vi "Dashboard custom_bartender&global&gripper.vi"() -> ()   [LabVIEW 2017]
uses:
  C:/Users/IMR Lab/Documents/LabVIEW Data/UniversalRobotsSDK_LABView/LabVIEW/Examples/LabVIEW10/UnderAutomation.UniversalRobots.dll
  UnderAutomation.UniversalRobots.dll
  Global 1.vi
panel:
  out "3rd Order":bool
  out "2nd Order":bool
  out "1st Order":bool
  in  "stop":bool
  in  "TCP switch (server)":bool
  out "Rx":dbl
  out "Rz":dbl
  out "Ry":dbl
  out "Enabled":bool
  out "Port":i32
  in  "Move to particular posture":bool
  in  "Move to Zero position":bool
  out "Connected":bool
  in  "Robot IP(192.168.112.182)":string
  out "Connect error":errorcluster
  in  "Power on\nRelease brake":bool
  in  "Power off":bool
  in  "Connect":bool
  in  "Send script":bool
  in  "Script to execute":string
  out "Powered on":bool
  out "X":dbl
  out "Y":dbl
  out "Z":dbl
  out "License state":string
  # "movel(p[-0.0753945, -0.304532, 0.314608, -0.194623, 2.71667, -1.00228], a= 0.5, v=0.25)"
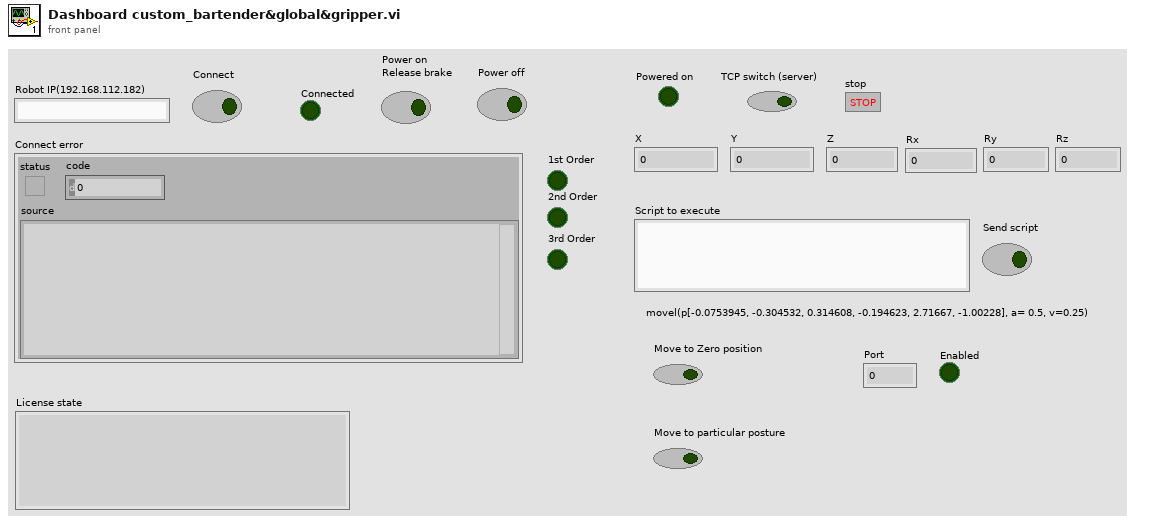
[diagram p1: front panel]
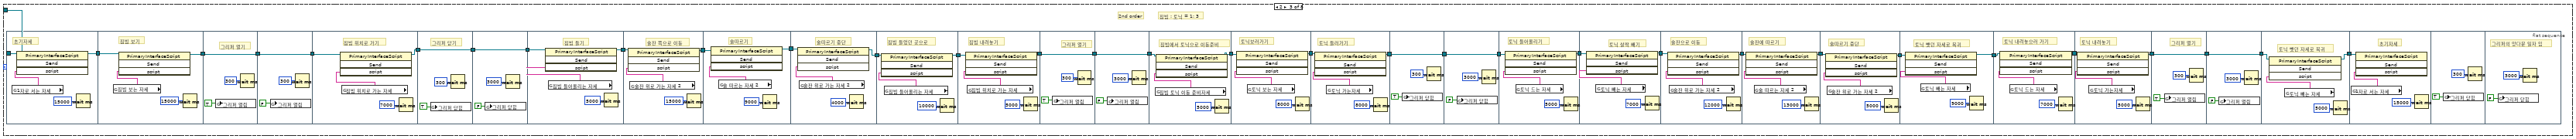
[diagram p5: hidden frame]
diagram:
  # "미니콜라 따르는 자세"
  # "술잔 중간지점 가는 자세"
  # "짐빔에서 토닉이동 준비 자세"
  # "술잔 따르는 자세2"
  # "술잔 위로 가는 자세2"
  # "토닉워터 뺴는 자세"
  # "토닉워 들어올리는 자세"
  # "토닉워터 가는 자세"
  # "토닉워터 보는 자세"
  # "짐빔 들어올리는 자세"
  # "짐빔로 가는 자세"
  # "짐빔 보는 자세"
  # "콜라 뺴는 자세"
  # "콜라 들어올리는 자세"
  # "콜라로 가는 자세"
  # "콜라 보는 자세"
  # "술잔 따르는 자세"
  # "술잔 위로 가는 자세"
  # "잭다니엘 들어올리는 자세"
  # "잭다니엘 위치로 가는 자세"
  # "잭다니엘 보는 자세"
  # "1자로 서는 자세"
  # "Example : Display power on status"
  # "Create a UR\ncobot instance"
  # "Show license state"
  # "Register your confidential license key to exit\ntrial period and use this library forever"
  # "Power off when button is clicked"
  # "Power on and release brake when button is clicked"
  # "Get your UR Dashboard interface"
  n1 = global write "Global 1.vi" "미니콜라 따르는 자세"("movej([-0.0902,-1.8120,-1.9241,-3.5769,6.2827,8.4658], a=0.5, v=0.25, t=0, r=0)") -> ()
  n2 = global write "Global 1.vi" "술잔 중간지점"("movej([-0.2173,-1.9485,-1.6874,-3.9352,6.2671,7.2276], a=0.5, v=0.25, t=0, r=0)") -> ()
  n3 = global write "Global 1.vi" "짐빔 토닉 이동 준비자세"("movej([-0.5421,-0.8131,0.8439,-0.0538,2.5052,5.9032], a=0.5, v=0.25, t=0, r=0)") -> ()
  n4 = global write "Global 1.vi" "잭다니엘 들어올리는 자세"("movej([0.8116,-2.0223,-1.2828,-3.0107,4.3284,5.9341], a=0.5, v=0.25, t=0, r=0)") -> ()
  n5 = global write "Global 1.vi" "잭다닐 위치로 가는 자세"("movej([0.8116,-2.3119,-1.606,-2.3958,4.3284,5.9341], a=0.5, v=0.25, t=0, r=0)") -> ()
  n6 = global write "Global 1.vi" "짐빔 들어올리는 자세"("movej([-0.5421,-0.8131,0.8439,-0.0538,2.5052,5.9032], a=0.5, v=0.25, t=0, r=0)") -> ()
  n7 = global write "Global 1.vi" "술잔 위로 가는 자세 2"("movej([0.0485,-1.6015,2.5780,-1.0382,-0.0520,5.3649], a=0.5, v=0.25, t=0, r=0)") -> ()
  n8 = global write "Global 1.vi" "1자로 서는 자세"("movej([3.1412,-1.5708,0,-1.5708,3.1412,5.8904], a=0.5, v=0.25, t=0, r=0)") -> ()
  n9 = global write "Global 1.vi" "짐빔 위치로 가는 자세"("movej([-0.5436,-0.4519,0.8428,-0.3534,2.6134,5.9032], a=0.5, v=0.25, t=0, r=0)") -> ()
  n10 = global write "Global 1.vi" "술잔 위로 가는 자세"("movej([-0.0903,-2.0548,-2.0169,-3.3289,6.2826,7.4091], a=0.5, v=0.25, t=0, r=0)") -> ()
  n11 = global write "Global 1.vi" "잭다니엘 보는 자세"("movej([0,-2.2170,-1.4226,-2.2842,3.1412,6.2832], a=0.5, v=0.25, t=0, r=0)") -> ()
  n12 = global write "Global 1.vi" "콜라 빼는 자세"("movej([0.8789,-1.5237,-2.1070,-2.6679, 3.9917,5.9085], a=0.5, v=0.25, t=0, r=0)") -> ()
  n13 = global write "Global 1.vi" "콜라 드는 자세"("movej([1.2020,-1.8452,-1.7403,-2.7082,4.3162,5.9158], a=0.5, v=0.25, t=0, r=0)") -> ()
  n14 = global write "Global 1.vi" "콜라 보는 자세"("movej([0,-1.8110,-2.1684,-2.3033,3.1543,5.9213], a=0.5, v=0.25, t=0, r=0)") -> ()
  n15 = global write "Global 1.vi" "콜라로 가는자세"("movej([1.2020,-2.166,-1.9385,-2.1863,4.3172,5.9210], a=0.5, v=0.25, t=0, r=0)") -> ()
  n16 = global write "Global 1.vi" "토닉 빼는 자세"("movej([-0.5277,-1.5104,1.5889,-0.0548,2.5728,5.9025], a=0.5, v=0.25, t=0, r=0)") -> ()
  n17 = global write "Global 1.vi" "술 따르는 자세 2"("movej([0.0412,-1.9708,2.4700,-1.0157,-0.0618,4.8998], a=0.5, v=0.25, t=0, r=0)") -> ()
  n18 = global write "Global 1.vi" "짐빔 보는 자세"("movej([-0.0364,-0.6154,0.9421,-0.3291,3.1047,5.9020], a=0.5, v=0.25, t=0, r=0)") -> ()
  n19 = global write "Global 1.vi" "토닉 드는 자세"("movej([-1.0311,-1.1460,1.5830,-0.4348,2.0708,5.9048], a=0.5, v=0.25, t=0, r=0)") -> ()
  n20 = global write "Global 1.vi" "토닉 보는 자세"("movej([-0.4690,-1.1292,2.1508,-1.0119,2.6124,5.9032], a=0.5, v=0.25, t=0, r=0)") -> ()
  n21 = global write "Global 1.vi" "술 따르는 자세"("movej([-0.0902,-1.9024,-1.9241,-3.5769,6.2827,8.4692], a=0.5, v=0.25, t=0, r=0)") -> ()
  n22 = global write "Global 1.vi" "토닉 가는자세"("movej([-0.9924,-0.8742,1.7459,-0.8837,2.0958,5.9048], a=0.5, v=0.25, t=0, r=0)") -> ()
  n23 = constructor class="UR"() -> (reference out=w25:refnum<k24>)  [unwired: 3 in, 2 out]
  n24 = while {
    tunnel: w25 -> [w31]
    stop <- FALSE stop-if-true
    # "Connect to the robot when button is pressed"
    # "Show if primary interface is connected"
    # "Get your UR primary interface"
    n25 = property class="UR"(reference=w31) -> ("PrimaryInterface"=w34:refnum<k24>)  [unwired: 1 in, 2 out]
    n26 = Wait (ms)(milliseconds to wait=u32 50) -> ()  [unwired: 1 out]
    n27 = property class="PrimaryInterfaceClientInternal"(reference=w34) -> ("Connected"=w33:bool)  [unwired: 1 in, 2 out]
    "Connected" <- w33
    n28 = case shown="True" "Connect" {
      tunnel: w31 -> [_ w397]
      frame False {
      }
      frame True {
        n29 = flat-sequence {
          tunnel: w397 -> [w399]
          frame #0 {
            n30 = invoke class="UR" method="Connect"(reference=w399, "ip"="Robot IP(192.168.112.182)") -> (error out=→"Connect error":errorcluster)  [unwired: 2 in, 3 out]
          }
        }
      }
    }
    n31 = case shown="True" w33 {
      tunnel: w34 -> [_ w55]
      frame False {
      }
      frame True {
        # "Send URScript when button pressed"
        # "Example : Display current cartesian pose"
        n32 = property class="PrimaryInterfaceClientInternal"(reference=w55) -> ("Script"=w40:refnum<k24>)  [unwired: 1 in, 2 out]
        n33 = global read "Global 1.vi" "2nd Order"() -> (w43:bool)
        "2nd Order" <- w43
        n34 = global read "Global 1.vi" "3rd Order"() -> (w42:bool)
        "3rd Order" <- w42
        n35 = global read "Global 1.vi" "1st Order"() -> (w44:bool)
        "1st Order" <- w44
        n36 = Build Array(w44, w43, w42) -> (w45:bool[])
        n37 = Boolean Array To Number(Boolean array=w45) -> (number=w41:u32)
        n38 = case shown="1" w41 {
          tunnel: w40 -> [_ w96 w232 _ _ _ _ _]
          frame 0, Default {
          }
          frame 1 {
            # "잭다 : 콜라 = 1 : 3"
            # "1st order"
            n39 = flat-sequence {
              tunnel: w96 -> [w100]
              tunnel: [w99] -> w95
              tunnel: w95 -> [w104]
              tunnel: [w102] -> w87
              tunnel: w87 -> [w107]
              tunnel: [w107] -> w85
              tunnel: w85 -> [w110]
              tunnel: [w110] -> w84
              tunnel: w84 -> [w114]
              tunnel: [w111] -> w86
              tunnel: w86 -> [w117]
              tunnel: [w117] -> w83
              tunnel: w83 -> [w120]
              tunnel: [w120] -> w82
              tunnel: w82 -> [w122]
              tunnel: [w121] -> w69
              tunnel: w69 -> [w126]
              tunnel: [w125] -> w68
              tunnel: w68 -> [w130]
              tunnel: [w129] -> w94
              tunnel: w94 -> [w135]
              tunnel: [w133] -> w93
              tunnel: w93 -> [w138]
              tunnel: [w137] -> w67
              tunnel: w67 -> [w142]
              tunnel: [w141] -> w66
              tunnel: [w145] -> w92
              tunnel: w66 -> [w147]
              tunnel: w92 -> [w150]
              tunnel: [w149] -> w81
              tunnel: w81 -> [w155]
              tunnel: [w155] -> w80
              tunnel: w80 -> [w158]
              tunnel: [w158] -> w79
              tunnel: w79 -> [w160]
              tunnel: [w159] -> w91
              tunnel: w91 -> [w164]
              tunnel: [w163] -> w78
              tunnel: w78 -> [w169]
              tunnel: [w169] -> w77
              tunnel: w77 -> [w172]
              tunnel: [w172] -> w76
              tunnel: w76 -> [w174]
              tunnel: [w173] -> w75
              tunnel: w75 -> [w178]
              tunnel: [w177] -> w65
              tunnel: w65 -> [w182]
              tunnel: [w181] -> w64
              tunnel: w64 -> [w186]
              tunnel: [w185] -> w90
              tunnel: w90 -> [w190]
              tunnel: [w189] -> w89
              tunnel: w89 -> [w194]
              tunnel: [w193] -> w63
              tunnel: w63 -> [w198]
              tunnel: [w197] -> w62
              tunnel: w62 -> [w202]
              tunnel: [w201] -> w74
              tunnel: w74 -> [w206]
              tunnel: [w205] -> w88
              tunnel: w88 -> [w210]
              tunnel: [w209] -> w72
              tunnel: [w213] -> w73
              tunnel: w72 -> [w213]
              tunnel: [w216] -> w71
              tunnel: w73 -> [w216]
              tunnel: w71 -> [w220]
              tunnel: [w219] -> w70
              tunnel: w70 -> [w223]
              frame #0 {
                # "초기자세"
                n40 = global read "Global 1.vi" "1자로 서는 자세"() -> (w98:string)
                n41 = invoke class="PrimaryInterfaceScript" method="Send"(reference=w100, "script"=w98) -> (reference out=w99:refnum<k24>)  [unwired: 2 in, 3 out]
                n42 = Wait (ms)(milliseconds to wait=u32 15000) -> ()  [unwired: 1 out]
              }
              frame #1 {
                # "잭다니엘 보기"
                n43 = global read "Global 1.vi" "잭다니엘 보는 자세"() -> (w103:string)
                n44 = invoke class="PrimaryInterfaceScript" method="Send"(reference=w104, "script"=w103) -> (reference out=w102:refnum<k24>)  [unwired: 2 in, 3 out]
                n45 = Wait (ms)(milliseconds to wait=u32 15000) -> ()  [unwired: 1 out]
              }
              frame #2 {
                # "그리퍼 열기"
                n46 = global write "Global 1.vi" "그리퍼 열림"(TRUE ("그리퍼 열림")) -> ()
                n47 = Wait (ms)(milliseconds to wait=u32 300) -> ()  [unwired: 1 out]
              }
              frame #3 {
                n48 = global write "Global 1.vi" "그리퍼 열림"(FALSE ("그리퍼 열림")) -> ()
                n49 = Wait (ms)(milliseconds to wait=u32 300) -> ()  [unwired: 1 out]
              }
              frame #4 {
                # "잭다니엘 위치로 가기"
                n50 = global read "Global 1.vi" "잭다닐 위치로 가는 자세"() -> (w113:string)
                n51 = invoke class="PrimaryInterfaceScript" method="Send"(reference=w114, "script"=w113) -> (reference out=w111:refnum<k24>)  [unwired: 2 in, 3 out]
                n52 = Wait (ms)(milliseconds to wait=u32 7000) -> ()  [unwired: 1 out]
              }
              frame #5 {
                # "그리퍼 닫기"
                n53 = global write "Global 1.vi" "그리퍼 닫힘"(TRUE ("그리퍼 열림")) -> ()
                n54 = Wait (ms)(milliseconds to wait=u32 300) -> ()  [unwired: 1 out]
              }
              frame #6 {
                n55 = global write "Global 1.vi" "그리퍼 닫힘"(FALSE ("그리퍼 열림")) -> ()
                n56 = Wait (ms)(milliseconds to wait=u32 3000) -> ()  [unwired: 1 out]
              }
              frame #7 {
                # "잭다니엘 들기"
                n57 = global read "Global 1.vi" "잭다니엘 들어올리는 자세"() -> (w124:string)
                n58 = invoke class="PrimaryInterfaceScript" method="Send"(reference=w122, "script"=w124) -> (reference out=w121:refnum<k24>)  [unwired: 2 in, 3 out]
                n59 = Wait (ms)(milliseconds to wait=u32 3000) -> ()  [unwired: 1 out]
              }
              frame #8 {
                # "술잔 중간지점으로 이동"
                n60 = global read "Global 1.vi" "술잔 중간지점"() -> (w127:string)
                n61 = invoke class="PrimaryInterfaceScript" method="Send"(reference=w126, "script"=w127) -> (reference out=w125:refnum<k24>)  [unwired: 2 in, 3 out]
                n62 = Wait (ms)(milliseconds to wait=u32 15000) -> ()  [unwired: 1 out]
              }
              frame #9 {
                # "술잔 쪽으로 이동"
                n63 = global read "Global 1.vi" "술잔 위로 가는 자세"() -> (w131:string)
                n64 = invoke class="PrimaryInterfaceScript" method="Send"(reference=w130, "script"=w131) -> (reference out=w129:refnum<k24>)  [unwired: 2 in, 3 out]
                n65 = Wait (ms)(milliseconds to wait=u32 5000) -> ()  [unwired: 1 out]
              }
              frame #10 {
                # "술따르기"
                n66 = global read "Global 1.vi" "술 따르는 자세"() -> (w134:string)
                n67 = invoke class="PrimaryInterfaceScript" method="Send"(reference=w135, "script"=w134) -> (reference out=w133:refnum<k24>)  [unwired: 2 in, 3 out]
                n68 = Wait (ms)(milliseconds to wait=u32 9000) -> ()  [unwired: 1 out]
              }
              frame #11 {
                # "술따르기 중단"
                n69 = global read "Global 1.vi" "술잔 위로 가는 자세"() -> (w139:string)
                n70 = invoke class="PrimaryInterfaceScript" method="Send"(reference=w138, "script"=w139) -> (reference out=w137:refnum<k24>)  [unwired: 2 in, 3 out]
                n71 = Wait (ms)(milliseconds to wait=u32 4000) -> ()  [unwired: 1 out]
              }
              frame #12 {
                # "술잔 중간지점으로 이동"
                n72 = global read "Global 1.vi" "술잔 중간지점"() -> (w143:string)
                n73 = invoke class="PrimaryInterfaceScript" method="Send"(reference=w142, "script"=w143) -> (reference out=w141:refnum<k24>)  [unwired: 2 in, 3 out]
                n74 = Wait (ms)(milliseconds to wait=u32 7000) -> ()  [unwired: 1 out]
              }
              frame #13 {
                # "잭다니엘 들었던 곳으로"
                n75 = global read "Global 1.vi" "잭다니엘 들어올리는 자세"() -> (w146:string)
                n76 = invoke class="PrimaryInterfaceScript" method="Send"(reference=w147, "script"=w146) -> (reference out=w145:refnum<k24>)  [unwired: 2 in, 3 out]
                n77 = Wait (ms)(milliseconds to wait=u32 10000) -> ()  [unwired: 1 out]
              }
              frame #14 {
                # "잭다니엘 내려놓기"
                n78 = global read "Global 1.vi" "잭다닐 위치로 가는 자세"() -> (w152:string)
                n79 = invoke class="PrimaryInterfaceScript" method="Send"(reference=w150, "script"=w152) -> (reference out=w149:refnum<k24>)  [unwired: 2 in, 3 out]
                n80 = Wait (ms)(milliseconds to wait=u32 5000) -> ()  [unwired: 1 out]
              }
              frame #15 {
                # "그리퍼 열기"
                n81 = global write "Global 1.vi" "그리퍼 열림"(TRUE ("그리퍼 열림")) -> ()
                n82 = Wait (ms)(milliseconds to wait=u32 300) -> ()  [unwired: 1 out]
              }
              frame #16 {
                n83 = global write "Global 1.vi" "그리퍼 열림"(FALSE ("그리퍼 열림")) -> ()
                n84 = Wait (ms)(milliseconds to wait=u32 3000) -> ()  [unwired: 1 out]
              }
              frame #17 {
                # "콜라보러가기"
                n85 = global read "Global 1.vi" "콜라 보는 자세"() -> (w162:string)
                n86 = invoke class="PrimaryInterfaceScript" method="Send"(reference=w160, "script"=w162) -> (reference out=w159:refnum<k24>)  [unwired: 2 in, 3 out]
                n87 = Wait (ms)(milliseconds to wait=u32 8000) -> ()  [unwired: 1 out]
              }
              frame #18 {
                # "콜라 들러가기"
                n88 = global read "Global 1.vi" "콜라로 가는자세"() -> (w166:string)
                n89 = invoke class="PrimaryInterfaceScript" method="Send"(reference=w164, "script"=w166) -> (reference out=w163:refnum<k24>)  [unwired: 2 in, 3 out]
                n90 = Wait (ms)(milliseconds to wait=u32 8000) -> ()  [unwired: 1 out]
              }
              frame #19 {
                n91 = global write "Global 1.vi" "그리퍼 닫힘"(TRUE ("그리퍼 열림")) -> ()
                n92 = Wait (ms)(milliseconds to wait=u32 300) -> ()  [unwired: 1 out]
              }
              frame #20 {
                n93 = global write "Global 1.vi" "그리퍼 닫힘"(FALSE ("그리퍼 열림")) -> ()
                n94 = Wait (ms)(milliseconds to wait=u32 3000) -> ()  [unwired: 1 out]
              }
              frame #21 {
                # "콜라 들어올리기"
                n95 = global read "Global 1.vi" "콜라 드는 자세"() -> (w176:string)
                n96 = invoke class="PrimaryInterfaceScript" method="Send"(reference=w174, "script"=w176) -> (reference out=w173:refnum<k24>)  [unwired: 2 in, 3 out]
                n97 = Wait (ms)(milliseconds to wait=u32 5000) -> ()  [unwired: 1 out]
              }
              frame #22 {
                # "콜라 살짝 빼기"
                n98 = global read "Global 1.vi" "콜라 빼는 자세"() -> (w180:string)
                n99 = invoke class="PrimaryInterfaceScript" method="Send"(reference=w178, "script"=w180) -> (reference out=w177:refnum<k24>)  [unwired: 2 in, 3 out]
                n100 = Wait (ms)(milliseconds to wait=u32 5000) -> ()  [unwired: 1 out]
              }
              frame #23 {
                # "술잔 중간지점으로 이동"
                n101 = global read "Global 1.vi" "술잔 중간지점"() -> (w183:string)
                n102 = invoke class="PrimaryInterfaceScript" method="Send"(reference=w182, "script"=w183) -> (reference out=w181:refnum<k24>)  [unwired: 2 in, 3 out]
                n103 = Wait (ms)(milliseconds to wait=u32 15000) -> ()  [unwired: 1 out]
              }
              frame #24 {
                # "술잔으로 이동"
                n104 = global read "Global 1.vi" "술잔 위로 가는 자세"() -> (w188:string)
                n105 = invoke class="PrimaryInterfaceScript" method="Send"(reference=w186, "script"=w188) -> (reference out=w185:refnum<k24>)  [unwired: 2 in, 3 out]
                n106 = Wait (ms)(milliseconds to wait=u32 5000) -> ()  [unwired: 1 out]
              }
              frame #25 {
                # "미니콜라에 따르기"
                n107 = global read "Global 1.vi" "미니콜라 따르는 자세"() -> (w192:string)
                n108 = invoke class="PrimaryInterfaceScript" method="Send"(reference=w190, "script"=w192) -> (reference out=w189:refnum<k24>)  [unwired: 2 in, 3 out]
                n109 = Wait (ms)(milliseconds to wait=u32 11000) -> ()  [unwired: 1 out]
              }
              frame #26 {
                # "술따르기 중단"
                n110 = global read "Global 1.vi" "술잔 위로 가는 자세"() -> (w196:string)
                n111 = invoke class="PrimaryInterfaceScript" method="Send"(reference=w194, "script"=w196) -> (reference out=w193:refnum<k24>)  [unwired: 2 in, 3 out]
                n112 = Wait (ms)(milliseconds to wait=u32 5000) -> ()  [unwired: 1 out]
              }
              frame #27 {
                # "술잔 중간지점으로 이동"
                n113 = global read "Global 1.vi" "술잔 중간지점"() -> (w199:string)
                n114 = invoke class="PrimaryInterfaceScript" method="Send"(reference=w198, "script"=w199) -> (reference out=w197:refnum<k24>)  [unwired: 2 in, 3 out]
                n115 = Wait (ms)(milliseconds to wait=u32 7000) -> ()  [unwired: 1 out]
              }
              frame #28 {
                # "콜라 뻇던 자세로 복귀"
                n116 = global read "Global 1.vi" "콜라 빼는 자세"() -> (w203:string)
                n117 = invoke class="PrimaryInterfaceScript" method="Send"(reference=w202, "script"=w203) -> (reference out=w201:refnum<k24>)  [unwired: 2 in, 3 out]
                n118 = Wait (ms)(milliseconds to wait=u32 7000) -> ()  [unwired: 1 out]
              }
              frame #29 {
                # "콜라 내려놓으러 가기"
                n119 = global read "Global 1.vi" "콜라 드는 자세"() -> (w208:string)
                n120 = invoke class="PrimaryInterfaceScript" method="Send"(reference=w206, "script"=w208) -> (reference out=w205:refnum<k24>)  [unwired: 2 in, 3 out]
                n121 = Wait (ms)(milliseconds to wait=u32 10000) -> ()  [unwired: 1 out]
              }
              frame #30 {
                # "콜라 내려놓기"
                n122 = global read "Global 1.vi" "콜라로 가는자세"() -> (w212:string)
                n123 = invoke class="PrimaryInterfaceScript" method="Send"(reference=w210, "script"=w212) -> (reference out=w209:refnum<k24>)  [unwired: 2 in, 3 out]
                n124 = Wait (ms)(milliseconds to wait=u32 5000) -> ()  [unwired: 1 out]
              }
              frame #31 {
                # "그리퍼 열기"
                n125 = global write "Global 1.vi" "그리퍼 열림"(TRUE ("그리퍼 열림")) -> ()
                n126 = Wait (ms)(milliseconds to wait=u32 300) -> ()  [unwired: 1 out]
              }
              frame #32 {
                n127 = global write "Global 1.vi" "그리퍼 열림"(FALSE ("그리퍼 열림")) -> ()
                n128 = Wait (ms)(milliseconds to wait=u32 3000) -> ()  [unwired: 1 out]
              }
              frame #33 {
                # "콜라 뻇던 자세로 복귀"
                n129 = global read "Global 1.vi" "콜라 빼는 자세"() -> (w221:string)
                n130 = invoke class="PrimaryInterfaceScript" method="Send"(reference=w220, "script"=w221) -> (reference out=w219:refnum<k24>)  [unwired: 2 in, 3 out]
                n131 = Wait (ms)(milliseconds to wait=u32 5000) -> ()  [unwired: 1 out]
              }
              frame #34 {
                # "초기자세"
                n132 = global read "Global 1.vi" "1자로 서는 자세"() -> (w225:string)
                n133 = invoke class="PrimaryInterfaceScript" method="Send"(reference=w223, "script"=w225) -> ()  [unwired: 2 in, 4 out]
                n134 = Wait (ms)(milliseconds to wait=u32 15000) -> ()  [unwired: 1 out]
              }
              frame #35 {
                n135 = global write "Global 1.vi" "그리퍼 닫힘"(TRUE ("그리퍼 열림")) -> ()
                n136 = Wait (ms)(milliseconds to wait=u32 300) -> ()  [unwired: 1 out]
              }
              frame #36 {
                # "그리퍼의 앙다문 일자 입"
                n137 = global write "Global 1.vi" "그리퍼 닫힘"(FALSE ("그리퍼 열림")) -> ()
                n138 = Wait (ms)(milliseconds to wait=u32 3000) -> ()  [unwired: 1 out]
              }
            }
          }
          frame 2 {
            # "짐빔 : 토닉 = 1: 3"
            # "2nd order"
            n139 = flat-sequence {
              tunnel: w232 -> [w265]
              tunnel: [w264] -> w261
              tunnel: w261 -> [w269]
              tunnel: [w267] -> w260
              tunnel: w260 -> [w272]
              tunnel: [w272] -> w259
              tunnel: w259 -> [w275]
              tunnel: [w275] -> w258
              tunnel: w258 -> [w279]
              tunnel: [w276] -> w257
              tunnel: w257 -> [w282]
              tunnel: [w282] -> w256
              tunnel: w256 -> [w285]
              tunnel: [w285] -> w255
              tunnel: w255 -> [w287]
              tunnel: [w286] -> w254
              tunnel: w254 -> [w291]
              tunnel: [w290] -> w253
              tunnel: w253 -> [w296]
              tunnel: [w294] -> w252
              tunnel: w252 -> [w299]
              tunnel: [w298] -> w251
              tunnel: w251 -> [w304]
              tunnel: [w302] -> w250
              tunnel: w250 -> [w307]
              tunnel: [w306] -> w249
              tunnel: w249 -> [w312]
              tunnel: [w312] -> w248
              tunnel: w248 -> [w315]
              tunnel: [w315] -> w231
              tunnel: w231 -> [w317]
              tunnel: [w316] -> w230
              tunnel: [w320] -> w247
              tunnel: w230 -> [w321]
              tunnel: w247 -> [w325]
              tunnel: [w324] -> w246
              tunnel: w246 -> [w330]
              tunnel: [w330] -> w245
              tunnel: w245 -> [w333]
              tunnel: [w333] -> w244
              tunnel: w244 -> [w335]
              tunnel: [w334] -> w243
              tunnel: w243 -> [w339]
              tunnel: [w338] -> w242
              tunnel: w242 -> [w343]
              tunnel: [w342] -> w241
              tunnel: w241 -> [w347]
              tunnel: [w346] -> w240
              tunnel: w240 -> [w351]
              tunnel: [w350] -> w239
              tunnel: w239 -> [w355]
              tunnel: [w354] -> w238
              tunnel: w238 -> [w359]
              tunnel: [w358] -> w237
              tunnel: w237 -> [w363]
              tunnel: [w362] -> w236
              tunnel: [w366] -> w235
              tunnel: w236 -> [w366]
              tunnel: [w369] -> w234
              tunnel: w235 -> [w369]
              tunnel: w234 -> [w373]
              tunnel: [w372] -> w233
              tunnel: w233 -> [w376]
              frame #0 {
                # "초기자세"
                n140 = global read "Global 1.vi" "1자로 서는 자세"() -> (w263:string)
                n141 = invoke class="PrimaryInterfaceScript" method="Send"(reference=w265, "script"=w263) -> (reference out=w264:refnum<k24>)  [unwired: 2 in, 3 out]
                n142 = Wait (ms)(milliseconds to wait=u32 15000) -> ()  [unwired: 1 out]
              }
              frame #1 {
                # "짐빔 보기"
                n143 = global read "Global 1.vi" "짐빔 보는 자세"() -> (w268:string)
                n144 = invoke class="PrimaryInterfaceScript" method="Send"(reference=w269, "script"=w268) -> (reference out=w267:refnum<k24>)  [unwired: 2 in, 3 out]
                n145 = Wait (ms)(milliseconds to wait=u32 15000) -> ()  [unwired: 1 out]
              }
              frame #2 {
                # "그리퍼 열기"
                n146 = global write "Global 1.vi" "그리퍼 열림"(TRUE ("그리퍼 열림")) -> ()
                n147 = Wait (ms)(milliseconds to wait=u32 300) -> ()  [unwired: 1 out]
              }
              frame #3 {
                n148 = global write "Global 1.vi" "그리퍼 열림"(FALSE ("그리퍼 열림")) -> ()
                n149 = Wait (ms)(milliseconds to wait=u32 300) -> ()  [unwired: 1 out]
              }
              frame #4 {
                # "짐빔 위치로 가기"
                n150 = global read "Global 1.vi" "짐빔 위치로 가는 자세"() -> (w278:string)
                n151 = invoke class="PrimaryInterfaceScript" method="Send"(reference=w279, "script"=w278) -> (reference out=w276:refnum<k24>)  [unwired: 2 in, 3 out]
                n152 = Wait (ms)(milliseconds to wait=u32 7000) -> ()  [unwired: 1 out]
              }
              frame #5 {
                # "그리퍼 닫기"
                n153 = global write "Global 1.vi" "그리퍼 닫힘"(TRUE ("그리퍼 열림")) -> ()
                n154 = Wait (ms)(milliseconds to wait=u32 300) -> ()  [unwired: 1 out]
              }
              frame #6 {
                n155 = global write "Global 1.vi" "그리퍼 닫힘"(FALSE ("그리퍼 열림")) -> ()
                n156 = Wait (ms)(milliseconds to wait=u32 3000) -> ()  [unwired: 1 out]
              }
              frame #7 {
                # "짐빔 들기"
                n157 = global read "Global 1.vi" "짐빔 들어올리는 자세"() -> (w289:string)
                n158 = invoke class="PrimaryInterfaceScript" method="Send"(reference=w287, "script"=w289) -> (reference out=w286:refnum<k24>)  [unwired: 2 in, 3 out]
                n159 = Wait (ms)(milliseconds to wait=u32 5000) -> ()  [unwired: 1 out]
              }
              frame #8 {
                # "술잔 쪽으로 이동"
                n160 = global read "Global 1.vi" "술잔 위로 가는 자세 2"() -> (w292:string)
                n161 = invoke class="PrimaryInterfaceScript" method="Send"(reference=w291, "script"=w292) -> (reference out=w290:refnum<k24>)  [unwired: 2 in, 3 out]
                n162 = Wait (ms)(milliseconds to wait=u32 15000) -> ()  [unwired: 1 out]
              }
              frame #9 {
                # "술따르기"
                n163 = global read "Global 1.vi" "술 따르는 자세 2"() -> (w295:string)
                n164 = invoke class="PrimaryInterfaceScript" method="Send"(reference=w296, "script"=w295) -> (reference out=w294:refnum<k24>)  [unwired: 2 in, 3 out]
                n165 = Wait (ms)(milliseconds to wait=u32 9000) -> ()  [unwired: 1 out]
              }
              frame #10 {
                # "술따르기 중단"
                n166 = global read "Global 1.vi" "술잔 위로 가는 자세 2"() -> (w300:string)
                n167 = invoke class="PrimaryInterfaceScript" method="Send"(reference=w299, "script"=w300) -> (reference out=w298:refnum<k24>)  [unwired: 2 in, 3 out]
                n168 = Wait (ms)(milliseconds to wait=u32 4000) -> ()  [unwired: 1 out]
              }
              frame #11 {
                # "짐빔 들었던 곳으로"
                n169 = global read "Global 1.vi" "짐빔 들어올리는 자세"() -> (w303:string)
                n170 = invoke class="PrimaryInterfaceScript" method="Send"(reference=w304, "script"=w303) -> (reference out=w302:refnum<k24>)  [unwired: 2 in, 3 out]
                n171 = Wait (ms)(milliseconds to wait=u32 10000) -> ()  [unwired: 1 out]
              }
              frame #12 {
                # "짐빔 내려놓기"
                n172 = global read "Global 1.vi" "짐빔 위치로 가는 자세"() -> (w309:string)
                n173 = invoke class="PrimaryInterfaceScript" method="Send"(reference=w307, "script"=w309) -> (reference out=w306:refnum<k24>)  [unwired: 2 in, 3 out]
                n174 = Wait (ms)(milliseconds to wait=u32 5000) -> ()  [unwired: 1 out]
              }
              frame #13 {
                # "그리퍼 열기"
                n175 = global write "Global 1.vi" "그리퍼 열림"(TRUE ("그리퍼 열림")) -> ()
                n176 = Wait (ms)(milliseconds to wait=u32 300) -> ()  [unwired: 1 out]
              }
              frame #14 {
                n177 = global write "Global 1.vi" "그리퍼 열림"(FALSE ("그리퍼 열림")) -> ()
                n178 = Wait (ms)(milliseconds to wait=u32 3000) -> ()  [unwired: 1 out]
              }
              frame #15 {
                # "짐빔에서 토닉으로 이동준비"
                n179 = global read "Global 1.vi" "짐빔 토닉 이동 준비자세"() -> (w319:string)
                n180 = invoke class="PrimaryInterfaceScript" method="Send"(reference=w317, "script"=w319) -> (reference out=w316:refnum<k24>)  [unwired: 2 in, 3 out]
                n181 = Wait (ms)(milliseconds to wait=u32 5000) -> ()  [unwired: 1 out]
              }
              frame #16 {
                # "토닉보러가기"
                n182 = global read "Global 1.vi" "토닉 보는 자세"() -> (w323:string)
                n183 = invoke class="PrimaryInterfaceScript" method="Send"(reference=w321, "script"=w323) -> (reference out=w320:refnum<k24>)  [unwired: 2 in, 3 out]
                n184 = Wait (ms)(milliseconds to wait=u32 8000) -> ()  [unwired: 1 out]
              }
              frame #17 {
                # "토닉 들러가기"
                n185 = global read "Global 1.vi" "토닉 가는자세"() -> (w327:string)
                n186 = invoke class="PrimaryInterfaceScript" method="Send"(reference=w325, "script"=w327) -> (reference out=w324:refnum<k24>)  [unwired: 2 in, 3 out]
                n187 = Wait (ms)(milliseconds to wait=u32 8000) -> ()  [unwired: 1 out]
              }
              frame #18 {
                n188 = global write "Global 1.vi" "그리퍼 닫힘"(TRUE ("그리퍼 열림")) -> ()
                n189 = Wait (ms)(milliseconds to wait=u32 300) -> ()  [unwired: 1 out]
              }
              frame #19 {
                n190 = global write "Global 1.vi" "그리퍼 닫힘"(FALSE ("그리퍼 열림")) -> ()
                n191 = Wait (ms)(milliseconds to wait=u32 3000) -> ()  [unwired: 1 out]
              }
              frame #20 {
                # "토닉 들어올리기"
                n192 = global read "Global 1.vi" "토닉 드는 자세"() -> (w337:string)
                n193 = invoke class="PrimaryInterfaceScript" method="Send"(reference=w335, "script"=w337) -> (reference out=w334:refnum<k24>)  [unwired: 2 in, 3 out]
                n194 = Wait (ms)(milliseconds to wait=u32 5000) -> ()  [unwired: 1 out]
              }
              frame #21 {
                # "토닉 살짝 빼기"
                n195 = global read "Global 1.vi" "토닉 빼는 자세"() -> (w341:string)
                n196 = invoke class="PrimaryInterfaceScript" method="Send"(reference=w339, "script"=w341) -> (reference out=w338:refnum<k24>)  [unwired: 2 in, 3 out]
                n197 = Wait (ms)(milliseconds to wait=u32 7000) -> ()  [unwired: 1 out]
              }
              frame #22 {
                # "술잔으로 이동"
                n198 = global read "Global 1.vi" "술잔 위로 가는 자세 2"() -> (w345:string)
                n199 = invoke class="PrimaryInterfaceScript" method="Send"(reference=w343, "script"=w345) -> (reference out=w342:refnum<k24>)  [unwired: 2 in, 3 out]
                n200 = Wait (ms)(milliseconds to wait=u32 12000) -> ()  [unwired: 1 out]
              }
              frame #23 {
                # "술잔에 따르기"
                n201 = global read "Global 1.vi" "술 따르는 자세 2"() -> (w349:string)
                n202 = invoke class="PrimaryInterfaceScript" method="Send"(reference=w347, "script"=w349) -> (reference out=w346:refnum<k24>)  [unwired: 2 in, 3 out]
                n203 = Wait (ms)(milliseconds to wait=u32 13000) -> ()  [unwired: 1 out]
              }
              frame #24 {
                # "술따르기 중단"
                n204 = global read "Global 1.vi" "술잔 위로 가는 자세 2"() -> (w353:string)
                n205 = invoke class="PrimaryInterfaceScript" method="Send"(reference=w351, "script"=w353) -> (reference out=w350:refnum<k24>)  [unwired: 2 in, 3 out]
                n206 = Wait (ms)(milliseconds to wait=u32 5000) -> ()  [unwired: 1 out]
              }
              frame #25 {
                # "토닉 뻇던 자세로 복귀"
                n207 = global read "Global 1.vi" "토닉 빼는 자세"() -> (w356:string)
                n208 = invoke class="PrimaryInterfaceScript" method="Send"(reference=w355, "script"=w356) -> (reference out=w354:refnum<k24>)  [unwired: 2 in, 3 out]
                n209 = Wait (ms)(milliseconds to wait=u32 9000) -> ()  [unwired: 1 out]
              }
              frame #26 {
                # "토닉 내려놓으러 가기"
                n210 = global read "Global 1.vi" "토닉 드는 자세"() -> (w361:string)
                n211 = invoke class="PrimaryInterfaceScript" method="Send"(reference=w359, "script"=w361) -> (reference out=w358:refnum<k24>)  [unwired: 2 in, 3 out]
                n212 = Wait (ms)(milliseconds to wait=u32 7000) -> ()  [unwired: 1 out]
              }
              frame #27 {
                # "토닉 내려놓기"
                n213 = global read "Global 1.vi" "토닉 가는자세"() -> (w365:string)
                n214 = invoke class="PrimaryInterfaceScript" method="Send"(reference=w363, "script"=w365) -> (reference out=w362:refnum<k24>)  [unwired: 2 in, 3 out]
                n215 = Wait (ms)(milliseconds to wait=u32 5000) -> ()  [unwired: 1 out]
              }
              frame #28 {
                # "그리퍼 열기"
                n216 = global write "Global 1.vi" "그리퍼 열림"(TRUE ("그리퍼 열림")) -> ()
                n217 = Wait (ms)(milliseconds to wait=u32 300) -> ()  [unwired: 1 out]
              }
              frame #29 {
                n218 = global write "Global 1.vi" "그리퍼 열림"(FALSE ("그리퍼 열림")) -> ()
                n219 = Wait (ms)(milliseconds to wait=u32 3000) -> ()  [unwired: 1 out]
              }
              frame #30 {
                # "토닉 뻇던 자세로 복귀"
                n220 = global read "Global 1.vi" "토닉 빼는 자세"() -> (w374:string)
                n221 = invoke class="PrimaryInterfaceScript" method="Send"(reference=w373, "script"=w374) -> (reference out=w372:refnum<k24>)  [unwired: 2 in, 3 out]
                n222 = Wait (ms)(milliseconds to wait=u32 5000) -> ()  [unwired: 1 out]
              }
              frame #31 {
                # "초기자세"
                n223 = global read "Global 1.vi" "1자로 서는 자세"() -> (w378:string)
                n224 = invoke class="PrimaryInterfaceScript" method="Send"(reference=w376, "script"=w378) -> ()  [unwired: 2 in, 4 out]
                n225 = Wait (ms)(milliseconds to wait=u32 15000) -> ()  [unwired: 1 out]
              }
              frame #32 {
                n226 = global write "Global 1.vi" "그리퍼 닫힘"(TRUE ("그리퍼 열림")) -> ()
                n227 = Wait (ms)(milliseconds to wait=u32 300) -> ()  [unwired: 1 out]
              }
              frame #33 {
                # "그리퍼의 앙다문 일자 입"
                n228 = global write "Global 1.vi" "그리퍼 닫힘"(FALSE ("그리퍼 열림")) -> ()
                n229 = Wait (ms)(milliseconds to wait=u32 3000) -> ()  [unwired: 1 out]
              }
            }
          }
          frame 3 {
            # "multi order"
          }
          frame 4 {
            # "짐빔 : 우유 = 1 : 3"
            # "3rd order"
          }
          frame 5 {
            # "multi order"
          }
          frame 6 {
            # "multi order"
          }
          frame 7 {
            # "multi order"
          }
        }
        n230 = case shown="True" "Move to Zero position" {
          tunnel: w40 -> [_ w386]
          frame False {
          }
          frame True {
            n231 = flat-sequence {
              tunnel: w386 -> [w388]
              frame #0 {
                n232 = invoke class="PrimaryInterfaceScript" method="Send"(reference=w388, "script"="movej([0,-1.570795,0,-1.570795,0,0], a=1.4, v=1.05, t=0, r=0)") -> ()  [unwired: 2 in, 4 out]
              }
            }
          }
        }
        n233 = case shown="True" "Move to particular posture" {
          tunnel: w40 -> [_ w383]
          frame False {
          }
          frame True {
            n234 = flat-sequence {
              tunnel: w383 -> [w385]
              frame #0 {
                n235 = invoke class="PrimaryInterfaceScript" method="Send"(reference=w385, "script"="movej([-1.5,-1.5,-2,-0.5,1.8,0], a=1.4, v=1.05, t=0, r=0)") -> ()  [unwired: 2 in, 4 out]
              }
            }
          }
        }
        n236 = case shown="True" "Send script" {
          tunnel: w40 -> [_ w389]
          frame False {
          }
          frame True {
            n237 = flat-sequence {
              tunnel: w389 -> [w391]
              frame #0 {
                n238 = invoke class="PrimaryInterfaceScript" method="Send"(reference=w391, "script"="Script to execute") -> ()  [unwired: 2 in, 4 out]
              }
            }
          }
        }
        n239 = property class="PrimaryInterfaceClientInternal"(reference=w55) -> ("RobotModeData"=w60:refnum<k24>)  [unwired: 1 in, 2 out]
        n240 = property class="PrimaryInterfaceClientInternal"(reference=w55) -> ("CartesianInfo"=w47:refnum<k24>)  [unwired: 1 in, 2 out]
        n241 = property class="RobotModeDataPackageEventArgs"(reference=w60) -> ("RobotPowerOn"=→"Powered on":bool)  [unwired: 1 in, 2 out]
        n242 = constructor class="SocketCommunicationServer"() -> (reference out=w52:refnum<k24>)  [unwired: 3 in, 2 out]
        n243 = property class="SocketCommunicationServer"(reference=w52) -> ("Enabled"=→"Enabled":bool)  [unwired: 1 in, 2 out]
        n244 = property class="SocketCommunicationServer"(reference=w52) -> ("Port"=→"Port":i32)  [unwired: 1 in, 2 out]
        n245 = property class="CartesianInfoPackageEventArgs"(reference=w47) -> ("Y"=→"Y":dbl)  [unwired: 1 in, 2 out]
        n246 = property class="CartesianInfoPackageEventArgs"(reference=w47) -> ("Ry"=→"Ry":dbl)  [unwired: 1 in, 2 out]
        n247 = property class="CartesianInfoPackageEventArgs"(reference=w47) -> ("Z"=→"Z":dbl)  [unwired: 1 in, 2 out]
        n248 = property class="CartesianInfoPackageEventArgs"(reference=w47) -> ("Rz"=→"Rz":dbl)  [unwired: 1 in, 2 out]
        n249 = property class="CartesianInfoPackageEventArgs"(reference=w47) -> ("X"=→"X":dbl)  [unwired: 1 in, 2 out]
        n250 = property class="CartesianInfoPackageEventArgs"(reference=w47) -> ("Rx"=→"Rx":dbl)  [unwired: 1 in, 2 out]
      }
    }
    n251 = property class="UR"(reference=w31) -> ("Dashboard"=w35:refnum<k24>)  [unwired: 1 in, 2 out]
    n252 = case shown="True" "Power off" {
      tunnel: w35 -> [_ w392]
      frame False {
      }
      frame True {
        n253 = flat-sequence {
          tunnel: w392 -> [w393]
          frame #0 {
            n254 = invoke class="DashboardClientInternal" method="PowerOff"(reference=w393) -> ()  [unwired: 2 in, 3 out]
          }
        }
      }
    }
    n255 = case shown="True" "Power on\nRelease brake" {
      tunnel: w35 -> [_ w394]
      frame False {
      }
      frame True {
        n256 = flat-sequence {
          tunnel: w394 -> [w396]
          frame #0 {
            n257 = invoke class="DashboardClientInternal" method="PowerOn"(reference=w396) -> (reference out=w395:refnum<k24>)  [unwired: 2 in, 2 out]
            n258 = invoke class="DashboardClientInternal" method="ReleaseBrake"(reference=w395) -> ()  [unwired: 2 in, 3 out]
          }
        }
      }
    }
  }
  n259 = invoke class="UR" method="RegisterLicense"(reference=w25, "licensee"="your company name", "key"="") -> (reference out=w27:refnum<k24>)  [unwired: 2 in, 4 out]
  n260 = control-ref of="Script to execute"() -> (w24:refnum<vi>)
  n261 = property class="Str"(reference=w24, "Value"="movej([-1.5,-1.5,-2,-0.5,1.8,0], a=1.4, v=1.05, t=0, r=0)") -> ()  [unwired: 1 in, 2 out]
  n262 = property class="UR"(reference=w27) -> ("LicenseInfo"=w26:refnum<k24>)  [unwired: 1 in, 2 out]
  n263 = invoke class="LicenseInfo" method="ToString"(reference=w26) -> ("ToString"=→"License state":string)  [unwired: 2 in, 2 out]
  n264 = while {
    stop <- "stop" stop-if-true
    n265 = case shown="True" "TCP switch (server)" {
      frame False {
      }
      frame True {
        w405 = ", "
        n266 = local read "Ry"() -> (w412:dbl)
        n267 = local read "Rz"() -> (w411:dbl)
        n268 = local read "Rx"() -> (w413:dbl)
        n269 = local read "Y"() -> (w415:dbl)
        n270 = local read "X"() -> (w416:dbl)
        n271 = local read "Z"() -> (w414:dbl)
        n272 = Number To Fractional String(number=w412) -> (F-format string=w406:string)  [unwired: 3 in]
        n273 = Number To Fractional String(number=w414) -> (F-format string=w408:string)  [unwired: 3 in]
        n274 = Number To Fractional String(number=w411) -> (F-format string=w404:string)  [unwired: 3 in]
        n275 = Number To Fractional String(number=w416) -> (F-format string=w410:string)  [unwired: 3 in]
        n276 = Number To Fractional String(number=w415) -> (F-format string=w409:string)  [unwired: 3 in]
        n277 = Number To Fractional String(number=w413) -> (F-format string=w407:string)  [unwired: 3 in]
        n278 = TCP Open Connection(address="localhost", remote port or service name=u16 8089) -> (connection ID=w420:refnum<k5>, error out=w419:errorcluster)  [unwired: 3 in]
        n279 = Concatenate Strings(w410, w405, w409, w405, w408, w405, w407, w405, w406, w405, w404) -> (w403:string)
        n280 = TCP Write(connection ID=w420, data in=w403, error in (no error)=w419) -> (connection ID out=w418:refnum<k5>, error out=w417:errorcluster)  [unwired: 1 in, 1 out]
        n281 = TCP Close Connection(connection ID=w418, error in (no error)=w417) -> ()  [unwired: 1 in, 2 out]
      }
    }
  }
